vi "Temperature to Speed of Sound.vi"(9 "Pressure (pascals)":dbl=101325.0 format="%0.3f", 10 "Humidity":dbl=60.0 format="%0.3f", 11 "Temperature":dbl format="%0.3f") -> (1 "Cramer Speed of Sound at Tc Humid Air (m/s)":dbl, 3 "Speed of Sound at Tc Dry Air (m/s)":dbl)   [LabVIEW 2019]
panel:
  out "Difference  (m/s)":dbl
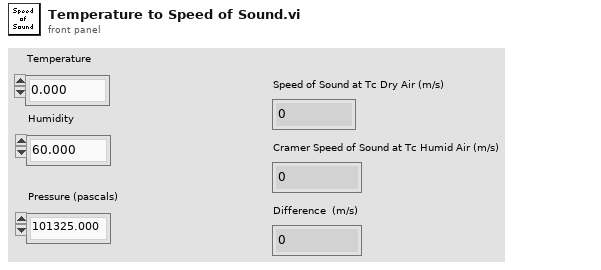
[diagram p1: front panel]
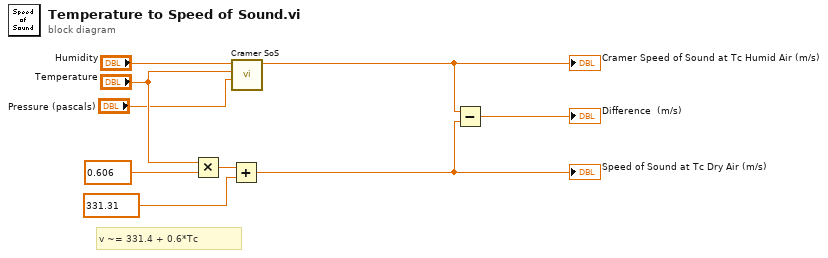
[diagram p0: block diagram]
diagram:
  # "v ~= 331.4 + 0.6*Tc"
  n1 = Multiply(x="Temperature", y=0.606) -> (x*y=w6:dbl)
  n2 = Add(x=w6, y=331.31) -> (x+y=w2:dbl)
  "Speed of Sound at Tc Dry Air (m/s)" <- w2
  n3 = call "Cramer SoS.vi"("Atmospheric pressure in Pa"="Pressure (pascals)", "Temperature"="Temperature", "Humidity"="Humidity") -> ("Cramer SoS"=w3:dbl)  [unwired: 8 in]
  "Cramer Speed of Sound at Tc Humid Air (m/s)" <- w3
  n4 = Subtract(x=w3, y=w2) -> (x-y=→"Difference  (m/s)":dbl)
